vi "DAQmx Create Channel (CI-Semi Period).vi"(0 "task in":refnum<k21>, 1 "maximum value":dbl=0.1 format="%.6f", 2 "minimum value":dbl=1e-06 format="%.6f", 5 "counter":tag, 7 "name to assign":string, 9 "units":i32(ring)=10364 items=["Seconds"=10364, "Ticks"=10304, "From Custom Scale"=10065], 11 "error in":errorcluster, 12 "custom scale name":tag) -> (4 "task out":refnum<k21>, 15 "error out":errorcluster)   [LabVIEW 2018]
doc: "Creates a channel to measure the time between state transitions of a digital signal. With the exception of devices that support multi-counter tasks, you can create only one counter input channel at a time with this VI because a task can contain only one counter input channel. To read from multiple counters simultaneously, use a separate task for each counter. Connect the input signal to the default input terminal of the counter unless you select a different input terminal."
uses:
  nilvaiu.dll
panel:
  # "input limits"
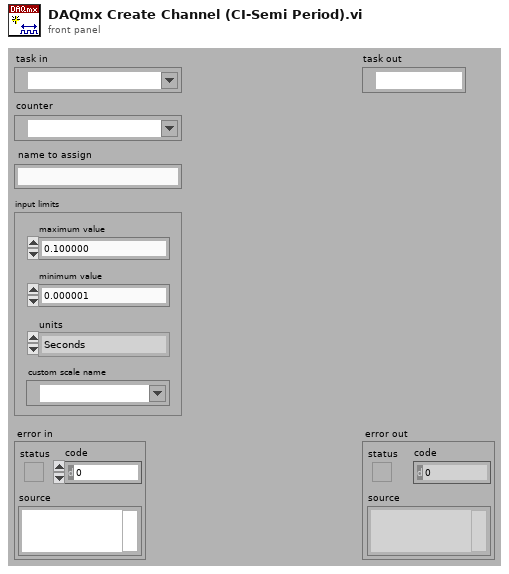
[diagram p1: front panel]
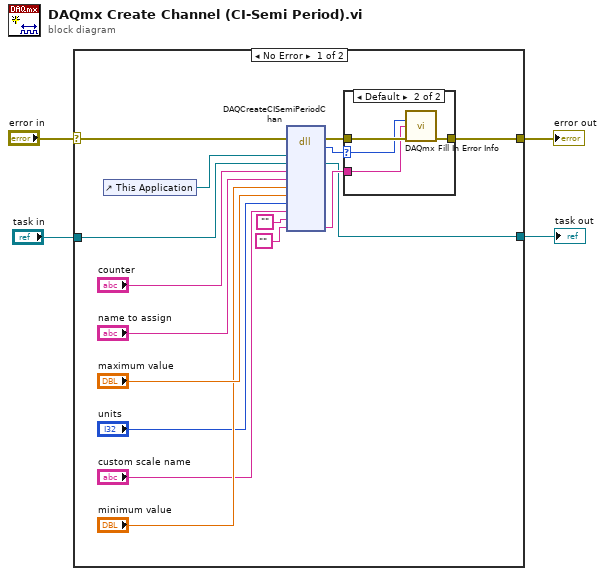
[diagram p0: block diagram]
diagram:
  n1 = case shown="No Error" "error in" {
    selector: "error in" -> [w6 w27]
    tunnel: [w9 w27] -> w4
    tunnel: "task in" -> [w8 w26]
    tunnel: [w7 w26] -> w2
    frame No Error {
      n2 = control-ref of="This Application"() -> (w17:refnum<vi>)
      n3 = dll-call lib="nilvaiu.*" fn="DAQCreateCISemiPeriodChan"(error in=w6, "lvAppRef"=w17, "refObjPtr"=w8, "counter"="counter", "channelNameIn"="name to assign", "minVal"="minimum value", "maxVal"="maximum value", "units"="units", "customScaleName"="custom scale name", "channelNamesOut"="", "extendedErrorInfo"="") -> (error out=w20:errorcluster, "return type"=w19:i32, "refObjPtr"=w7:refnum<k21>, "extendedErrorInfo"=w18:string)  [unwired: 10 in, 1 out]
      n4 = case shown="Default" w19 {
        selector: w19 -> [_ w23]
        tunnel: w20 -> [w21 w25]
        tunnel: [w21 w24] -> w9
        tunnel: w18 -> [_ w22]
        frame 0 {
        }
        frame Default {
          n5 = call "DAQmx Fill In Error Info.vi"("status code"=w23, "extended error info"=w22, "error in"=w25) -> ("error out"=w24:errorcluster)  [unwired: 1 in, 11 out]
        }
      }
    }
    frame Error {
    }
  }
  "error out" <- w4
  "task out" <- w2
